vi "DSF.Engine.Pointer.VS Channels.Set Channel Count.vi"(8 "error in (no error)":errorcluster, 10 "channel count":u64 format="%d channels", 11 "VS Channels Pointer in":refnum<class "DSF.Engine.Pointer.VS Channels.lvclass">) -> (0 "error out":errorcluster, 3 "VS Channels Pointer out":refnum<class "DSF.Engine.Pointer.VS Channels.lvclass">)   [LabVIEW 2016, in "DSF.Engine.lvlib" / "DSF.Engine.Pointer.VS Channels.lvclass"]
uses:
  DSF.Engine.Pointer.VS Channels.lvclass
  DSF.Engine.Pointer.VS Channels.lvclass/DSF.Engine.Pointer.VS Channels.ctl
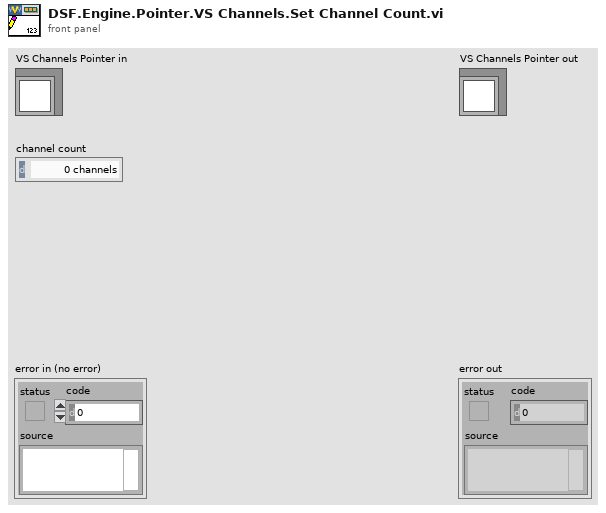
[diagram p1: front panel]
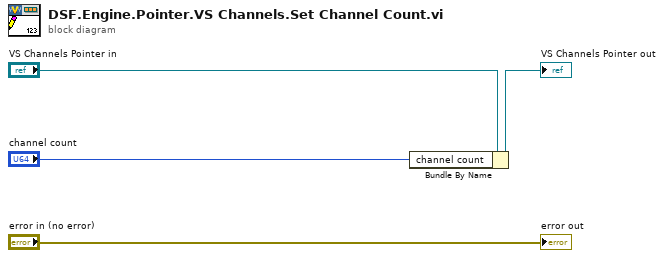
[diagram p0: block diagram]
diagram:
  n1 = Bundle By Name(cluster="VS Channels Pointer in", "channel count"="channel count") -> (→"VS Channels Pointer out":refnum<class "DSF.Engine.Pointer.VS Channels.lvclass">)
  "error out" <- "error in (no error)"
